vi "Untitled 5.vi"() -> ()   [LabVIEW 2023]
panel:
  out "B":i32
  out "A":i32
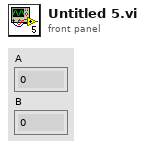
[diagram p1: front panel]
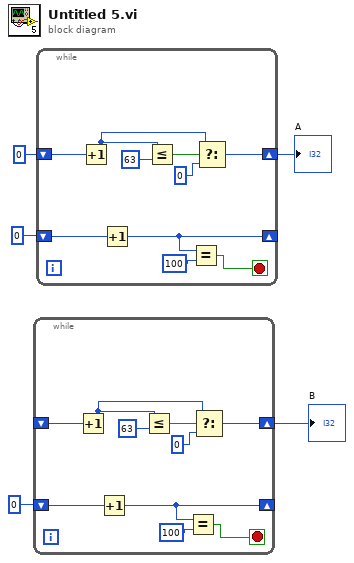
[diagram p0: block diagram]
diagram:
  n1 = while {
    shift-right: [w15] -> w1
    shift-left: _ -> [w10]
    shift-right: [w13] -> _
    shift-left: 0 -> [w14]
    stop <- w11 stop-if-true
    n2 = Increment(x=w10) -> (x+1=w8:i32)
    n3 = Increment(x=w14) -> (x+1=w13:i32)
    n4 = Less Or Equal?(x=w8, y=63) -> (x <= y?=w9:bool)
    n5 = Equal?(x=w13, y=100) -> (x = y?=w11:bool)
    n6 = Select(t=w8, s=w9, f=0) -> (s? t:f=w15:i32)
  }
  "B" <- w1
  n7 = while {
    shift-right: [w25] -> w2
    shift-left: 0 -> [w20]
    shift-right: [w23] -> _
    shift-left: 0 -> [w24]
    stop <- w21 stop-if-true
    n8 = Increment(x=w20) -> (x+1=w18:i32)
    n9 = Increment(x=w24) -> (x+1=w23:i32)
    n10 = Less Or Equal?(x=w18, y=63) -> (x <= y?=w19:bool)
    n11 = Equal?(x=w23, y=100) -> (x = y?=w21:bool)
    n12 = Select(t=w18, s=w19, f=0) -> (s? t:f=w25:i32)
  }
  "A" <- w2
